vi "in time.vi"() -> ()   [LabVIEW 2017]
panel:
  in  "in time 23":string
  in  "in time 22":string
  in  "in time 21":string
  in  "in time 20":string
  in  "in time 19":string
  in  "in time 18":string
  in  "in time 17":string
  in  "in time 16":string
  in  "in time 15":string
  in  "in time 14":string
  in  "in time 13":string
  in  "in time 12":string
  in  "in time 11":string
  in  "in time 10":string
  in  "in time 9":string
  in  "in time 8":string
  in  "in time 1":string
  in  "in time 2":string
  in  "in time 3":string
  in  "in time 7":string
  in  "in time 6":string
  in  "in time 5":string
  in  "in time 4":string
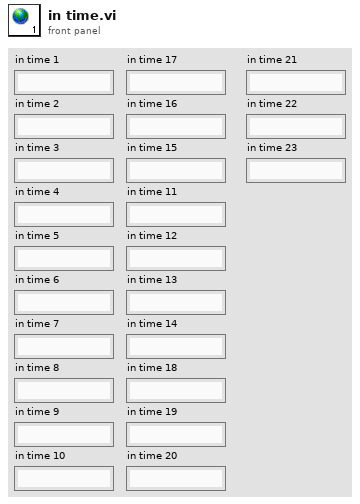
[diagram p1: front panel]
diagram:
